vi "Rigol_Scope_Configure_DS1102E.vi"(8 "error in (no error)":errorcluster, 11 "VISA resource name":refnum<visa-resource-name>="USB0::0x1AB1::0x0488::DS1BA202100064::INSTR") -> (0 "error out":errorcluster, 3 "VISA resource name out":refnum<visa-resource-name>)   [LabVIEW 2018]
uses:
  <vilib>/Utility/error.llb/DialogType.ctl
  <instrlib>/RIGOL DS1000 Series/RIGOL DS1000 Series.lvlib
panel:
  out "offsetV":string
  out "offsetT":string
  in  "offsetVoltage":dbl format="%#_6f"
  in  "offsetTime":dbl format="%#_6f"
  out "Command sent":string
  out "chann":string
  out "attn":string
  out "scaleT":string
  out "scaleV":string
  out "bandwidth":string
  out "triggerV":string
  out "filter":string
  in  "F Selector":bool=TRUE
  in  "triggerVoltage":dbl=0.5
  in  "Trigger Type (0: Edge)":u16(ring) items=["Edge", "Pulse", "Video", "Pattern", "Duration"]
  in  "scaleTime":dbl=0.001 format="%#_6f"
  in  "scaleVoltage":dbl=5.0
  in  "BW Selector":bool=TRUE
  in  "Vertical Coupling (0: DC)":u16(ring) items=["DC", "AC", "Ground"]
  in  "Attenuation":i32=1
  in  "Channel (0: Channel 1)":u16(ring) items=["Channel 1", "Channel 2", "Channel 3", "Channel 4"]
  # "Horizontal"
  # "Probe"
  # "Vertical"
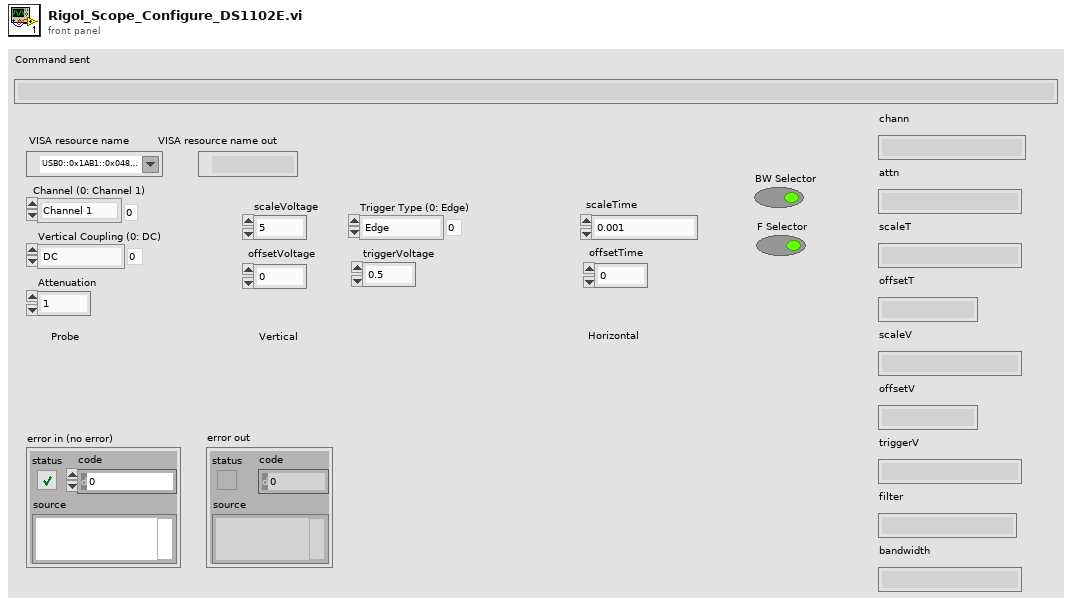
[diagram p1: front panel]
types:
  T1 = typedef "DialogType.ctl" = u16
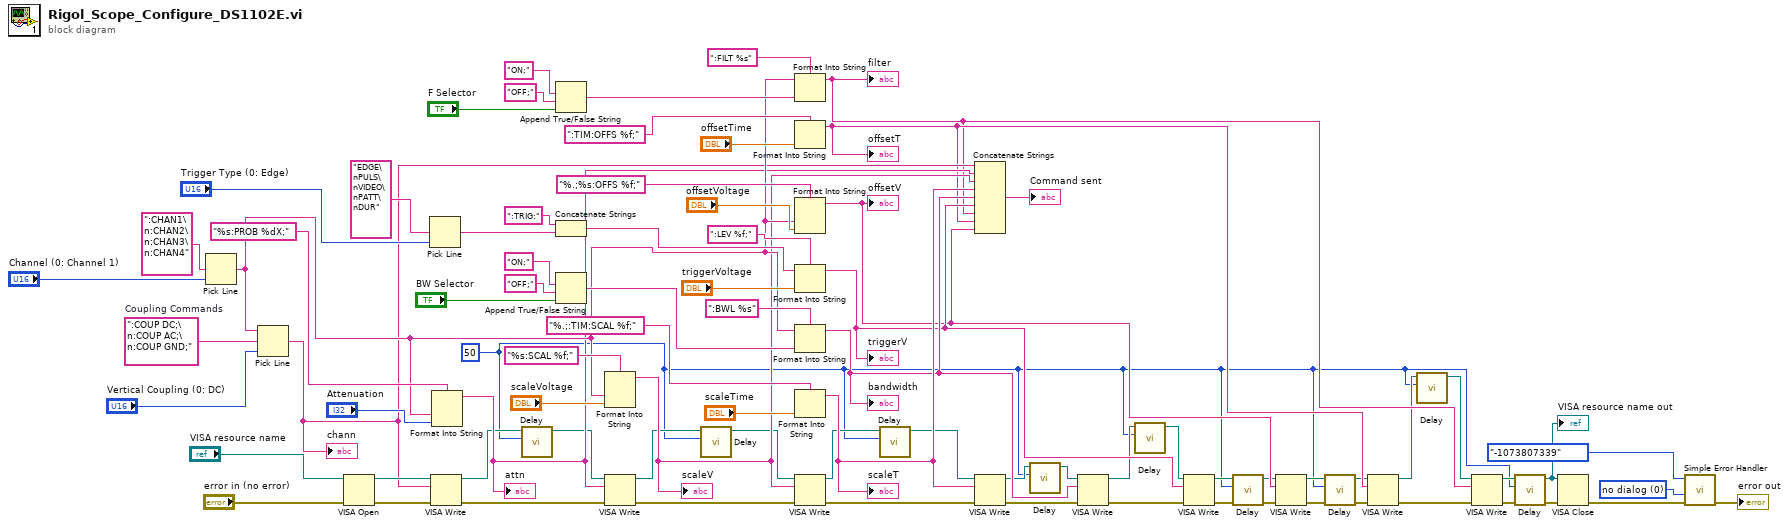
[diagram p0: block diagram]
diagram:
  w7 = u32 50 ("Delay (ms)")
  w48 = T1 0 items=["no dialog", "OK message", "continue or stop message", "OK message + warnings", "continue/stop + warnings"] ("type of dialog (OK msg:1)")
  w73 = ":COUP DC;\n:COUP AC;\n:COUP GND;"  # Coupling Commands
  n1 = Pick Line(multi-line string=":CHAN1\n:CHAN2\n:CHAN3\n:CHAN4" ("多行字符串"), line index="Channel (0: Channel 1)") -> (output string=w41:string)  [unwired: 1 out]
  n2 = Pick Line(string ("")=w41, multi-line string=w73, line index="Vertical Coupling (0: DC)") -> (output string=w40:string)
  "chann" <- w40
  n3 = VISA Open(error in (no error)="error in (no error)", VISA resource name="VISA resource name") -> (VISA resource name=w51:refnum<visa-resource-name>, error out=w52:errorcluster)  [unwired: 3 in]
  n4 = Pick Line(multi-line string="EDGE\nPULS\nVIDEO\nPATT\nDUR", line index="Trigger Type (0: Edge)") -> (output string=w66:string)  [unwired: 1 out]
  n5 = VISA Write(VISA resource name=w51, write buffer=w40, error in (no error)=w52) -> (VISA resource name out=w23:refnum<visa-resource-name>, error out=w26:errorcluster)  [unwired: 1 out]
  n6 = Format Into String(format string="%s:PROB %dX;", w41, "Attenuation") -> (resulting string=w39:string)  [unwired: 2 in, 1 out]
  "attn" <- w39
  n7 = call <instrlib>:"Delay.vi"("Delay (ms)"=w7, "VISA resource name"=w23) -> ("VISA resource name out"=w22:refnum<visa-resource-name>)  [unwired: 8 in, 1 out]
  n8 = Append True/False String(1:"F Selector", 2:"OFF;" ("false string"), 3:"ON;" ("true string")) -> (0:w56:string)  [unwired: 1 out]
  n9 = Concatenate Strings(":TRIG:" ("string (\"\")"), w66) -> (w60:string)
  n10 = Append True/False String(1:"BW Selector", 2:"OFF;" ("false string"), 3:"ON;" ("true string")) -> (0:w70:string)  [unwired: 1 out]
  n11 = Format Into String(format string="%s:SCAL %f;", w41, "scaleVoltage") -> (resulting string=w38:string)  [unwired: 2 in, 1 out]
  "scaleV" <- w38
  n12 = VISA Write(VISA resource name=w22, write buffer=w39, error in (no error)=w26) -> (VISA resource name out=w21:refnum<visa-resource-name>, error out=w32:errorcluster)  [unwired: 1 out]
  n13 = call <instrlib>:"Delay.vi"("Delay (ms)"=w7, "VISA resource name"=w21) -> ("VISA resource name out"=w20:refnum<visa-resource-name>)  [unwired: 8 in, 1 out]
  n14 = Format Into String(format string=":FILT %s", initial string=w41, w56) -> (resulting string=w24:string)  [unwired: 1 in, 1 out]
  "filter" <- w24
  n15 = Format Into String(format string=":TIM:OFFS %f;", "offsetTime") -> (resulting string=w33:string)  [unwired: 2 in, 1 out]
  "offsetT" <- w33
  n16 = Format Into String(format string="%.;%s:OFFS %f;", w41, "offsetVoltage") -> (resulting string=w25:string)  [unwired: 2 in, 1 out]
  "offsetV" <- w25
  n17 = Format Into String(format string=":LEV %f;", initial string=w60, "triggerVoltage") -> (resulting string=w34:string)  [unwired: 1 in, 1 out]
  "triggerV" <- w34
  n18 = Format Into String(format string=":BWL %s", initial string=w41, w70) -> (resulting string=w36:string)  [unwired: 1 in, 1 out]
  "bandwidth" <- w36
  n19 = Format Into String(format string="%.;:TIM:SCAL %f;", "scaleTime") -> (resulting string=w37:string)  [unwired: 2 in, 1 out]
  "scaleT" <- w37
  n20 = VISA Write(VISA resource name=w20, write buffer=w38, error in (no error)=w32) -> (VISA resource name out=w19:refnum<visa-resource-name>, error out=w31:errorcluster)  [unwired: 1 out]
  n21 = call <instrlib>:"Delay.vi"("Delay (ms)"=w7, "VISA resource name"=w19) -> ("VISA resource name out"=w18:refnum<visa-resource-name>)  [unwired: 8 in, 1 out]
  n22 = Concatenate Strings(w40, w39, w38, w37, w36, w34, w24, w33, w25) -> (→"Command sent":string)
  n23 = VISA Write(VISA resource name=w18, write buffer=w37, error in (no error)=w31) -> (VISA resource name out=w17:refnum<visa-resource-name>, error out=w30:errorcluster)  [unwired: 1 out]
  n24 = call <instrlib>:"Delay.vi"("Delay (ms)"=w7, "VISA resource name"=w17) -> ("VISA resource name out"=w16:refnum<visa-resource-name>)  [unwired: 8 in, 1 out]
  n25 = VISA Write(VISA resource name=w16, write buffer=w36, error in (no error)=w30) -> (VISA resource name out=w15:refnum<visa-resource-name>, error out=w29:errorcluster)  [unwired: 1 out]
  n26 = call <instrlib>:"Delay.vi"("Delay (ms)"=w7, "VISA resource name"=w15) -> ("VISA resource name out"=w14:refnum<visa-resource-name>)  [unwired: 8 in, 1 out]
  n27 = VISA Write(VISA resource name=w14, write buffer=w34, error in (no error)=w29) -> (VISA resource name out=w13:refnum<visa-resource-name>, error out=w4:errorcluster)  [unwired: 1 out]
  n28 = call <instrlib>:"Delay.vi"("error in (no error)"=w4, "Delay (ms)"=w7, "VISA resource name"=w13) -> ("error out"=w3:errorcluster, "VISA resource name out"=w12:refnum<visa-resource-name>)  [unwired: 7 in]
  n29 = VISA Write(VISA resource name=w12, write buffer=w25, error in (no error)=w3) -> (VISA resource name out=w11:refnum<visa-resource-name>, error out=w2:errorcluster)  [unwired: 1 out]
  n30 = call <instrlib>:"Delay.vi"("error in (no error)"=w2, "Delay (ms)"=w7, "VISA resource name"=w11) -> ("error out"=w1:errorcluster, "VISA resource name out"=w10:refnum<visa-resource-name>)  [unwired: 7 in]
  n31 = VISA Write(VISA resource name=w10, write buffer=w33, error in (no error)=w1) -> (VISA resource name out=w9:refnum<visa-resource-name>, error out=w28:errorcluster)  [unwired: 1 out]
  n32 = call <instrlib>:"Delay.vi"("Delay (ms)"=w7, "VISA resource name"=w9) -> ("VISA resource name out"=w8:refnum<visa-resource-name>)  [unwired: 8 in, 1 out]
  n33 = VISA Write(VISA resource name=w8, write buffer=w24, error in (no error)=w28) -> (VISA resource name out=w35:refnum<visa-resource-name>, error out=w27:errorcluster)  [unwired: 1 out]
  n34 = call <instrlib>:"Delay.vi"("error in (no error)"=w27, "Delay (ms)"=w7, "VISA resource name"=w35) -> ("error out"=w49:errorcluster, "VISA resource name out"=w50:refnum<visa-resource-name>)  [unwired: 7 in]
  "VISA resource name out" <- w50
  n35 = VISA Close(VISA resource name=w50, error in (no error)=w49) -> (error out=w46:errorcluster)
  n36 = call <vilib>:"Simple Error Handler.vi"("error code (no error:0)"=enum16{"-1073807339"}."-1073807339", "type of dialog (OK msg:1)"=w48, "error in (no error)"=w46) -> ("error out"=→"error out":errorcluster)  [unwired: 2 in, 4 out]
